vi "MockDisplacement.vi"(11 "MockDisplacementSettings":T1={"SerialPort"="Slot3\\Port1", "BufferUpdateFIFO"="MockDisplacementCommandFIFO", "DisplacementMemory"="DisplacementMemory"}) -> ()   [LabVIEW 2016, in "FPGAMockDisplacement.lvlib"]
uses:
  FPGAMockDisplacement.lvlib
  DataTypes/MockDisplacementSettings.ctl
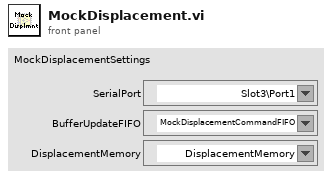
[diagram p1: front panel]
types:
  T1 = typedef "FPGAMockDisplacement.lvlib/MockDisplacementSettings.ctl" = cluster{"SerialPort":refnum<k21>, "BufferUpdateFIFO":refnum<k21>, "DisplacementMemory":refnum<k21>}
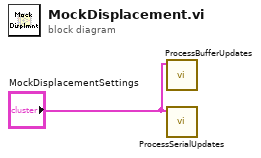
[diagram p0: block diagram]
diagram:
  n1 = call "ProcessBufferUpdates.vi"("MockDisplacementSettings"="MockDisplacementSettings") -> ()  [unwired: 11 in]
  n2 = call "ProcessSerialUpdates.vi"("MockDisplacementSettings"="MockDisplacementSettings") -> ()  [unwired: 11 in]
